vi "oa_Extract XY Signal Segment (2D Array).vi"(0 "XY signals":cluster{"X":dbl[], "Y":dbl[]}[][](array[cluster]) {"X" format="%.2f"; "Y" format="%.2f"}, 1 "X axis selection":u16(ring)=2 items=["Time", "Revolution", "RPM"], 2 "reset? (F)":bool, 5 "trigger indices":T1, 7 "position info in":T2, 11 "error in (no error)":errorcluster, 12 "indices end?":bool) -> (4 "XY signals out":cluster{"X":dbl[], "Y":dbl[]}[][](array[cluster]) {"X" format="%.2f"; "Y" format="%.2f"}, 8 "position info out":T2, 14 "reached end?":bool, 15 "error out":errorcluster)   [LabVIEW 2017, in "SoundVib_OAUtility.lvlib"]
uses:
  <vilib>/addons/Sound and Vibration/Order Analysis/Utility/SoundVib_OAUtility.lvlib
  <vilib>/addons/Sound and Vibration/Order Analysis/Misc/OAT Position Info.ctl
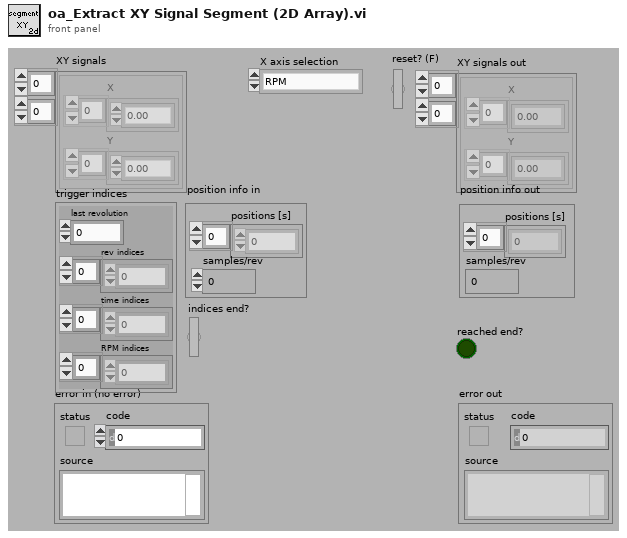
[diagram p1: front panel]
types:
  T1 = cluster{"last revolution":dbl, "rev indices":dbl[], "time indices":dbl[], "RPM indices":dbl[]}
  T2 = typedef "OAT Position Info.ctl" = cluster{"positions [s]":dbl[], "samples/rev":dbl}
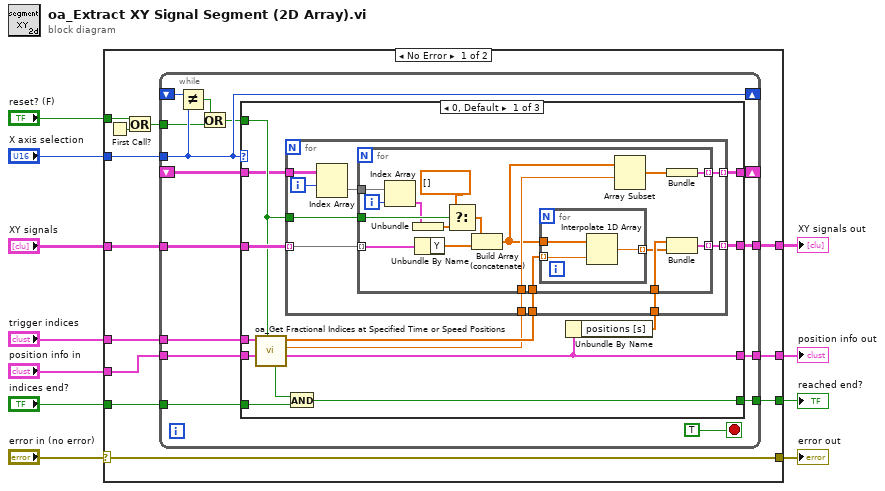
[diagram p0: block diagram]
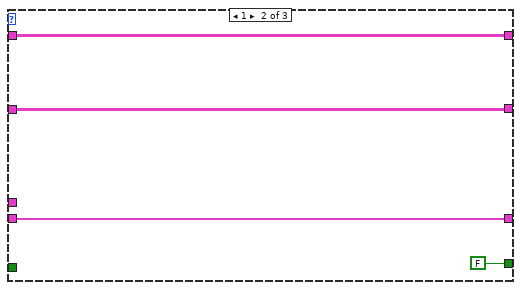
[diagram p2: hidden frame]
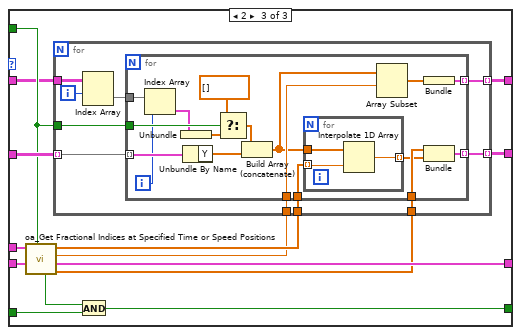
[diagram p3: hidden frame]
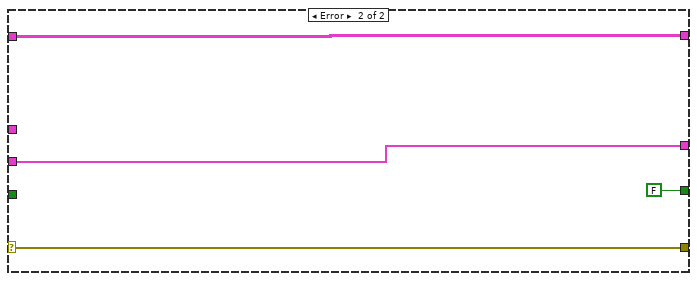
[diagram p4: hidden frame]
diagram:
  n1 = case shown="No Error" "error in (no error)" {
    selector: "error in (no error)" -> [w14 w134]
    tunnel: [w14 w134] -> w10
    tunnel: "reset? (F)" -> [w23 _]
    tunnel: "XY signals" -> [w19 w133]
    tunnel: [w20 w133] -> w7
    tunnel: "position info in" -> [w16 w132]
    tunnel: "trigger indices" -> [w17 _]
    tunnel: "X axis selection" -> [w21 _]
    tunnel: [w15 w132] -> w3
    tunnel: "indices end?" -> [w13 _]
    tunnel: [w12 FALSE] -> w1
    frame No Error {
      n2 = First Call?() -> (First Call?: T/F=w22:bool)
      n3 = Or(x=w23, y=w22) -> (x .or. y?=w18:bool)
      n4 = while {
        tunnel: w21 -> [w29]
        tunnel: [w38] -> w20
        tunnel: w19 -> [w37]
        tunnel: w18 -> [w27]
        tunnel: w17 -> [w36]
        tunnel: w16 -> [w35]
        tunnel: [w34] -> w15
        shift-right: [w32] -> _
        shift-left: _ -> [w31]
        shift-right: [w29] -> _
        shift-left: _ -> [w30]
        tunnel: w13 -> [w25]
        tunnel: [w24] -> w12
        stop <- TRUE stop-if-true
        n5 = Not Equal?(x=w30, y=w29) -> (x != y?=w26:bool)
        n6 = Or(x=w26, y=w27) -> (x .or. y?=w28:bool)
        n7 = case shown="0, Default" w29 {
          tunnel: [w46 w86 w95] -> w38
          tunnel: w37 -> [w50 w86 w98]
          tunnel: w28 -> [w43 _ w97]
          tunnel: w36 -> [w52 _ w94]
          tunnel: w35 -> [w51 w85 w93]
          tunnel: [w48 w85 w92] -> w34
          tunnel: [w44 w84 w96] -> w32
          tunnel: w31 -> [w42 w84 w90]
          tunnel: w25 -> [w41 _ w89]
          tunnel: [w39 FALSE w87] -> w24
          frame 0, Default {
            n8 = call <vilib>:"oa_Get Fractional Indices at Specified Time or Speed Positions.vi"("reset? (F)"=w43, "position info in"=w51, "trigger indices"=w52) -> ("position info out"=w48:T2, "buffer index"=w45:dbl, "fractional indices out"=w49:dbl[], "indices buffer empty?"=w40:bool)  [unwired: 4 in, 1 out]
            n9 = And(x=w40, y=w41) -> (x .and. y?=w39:bool)
            n10 = Unbundle By Name(w48) -> ("positions [s]"=w47:dbl[])
            n11 = for {
              tunnel: w50 -> [w62] mode=indexing
              tunnel: w49 -> [w61]
              tunnel: w47 -> [w60]
              tunnel: [w59] -> w46 mode=indexing
              tunnel: w45 -> [w58]
              tunnel: [w57] -> w44 mode=indexing
              tunnel: w43 -> [w56]
              tunnel: w42 -> [w55]
              i -> [w54]
              n12 = Index Array(array=w55, index (row)=w54) -> (element=w53:cluster{dbl[]}[])  [unwired: 1 in]
              n13 = for {
                tunnel: w62 -> [w79] mode=indexing
                tunnel: w61 -> [w78]
                tunnel: w60 -> [w77]
                tunnel: [w76] -> w59 mode=indexing
                tunnel: w58 -> [w75]
                tunnel: [w74] -> w57 mode=indexing
                tunnel: w56 -> [w73]
                tunnel: w53 -> [w65]
                i -> [w63]
                n14 = Index Array(array=w65, index=w63) -> (element=w64:cluster{dbl[]})
                n15 = Unbundle(w64) -> (w70:dbl[])
                n16 = Unbundle By Name(w79) -> ("Y"=w68:dbl[])
                n17 = Select(t=dbl[] [], s=w73, f=w70) -> (s? t:f=w69:dbl[])
                n18 = Build Array (concatenate)(w69, w68) -> (w67:dbl[])
                n19 = for {
                  tunnel: w67 -> [w82]
                  tunnel: w78 -> [w81] mode=indexing
                  tunnel: [w80] -> w72 mode=indexing
                  n20 = Interpolate 1D Array(1:w81, 2:w82) -> (0:w80:dbl)
                }
                n21 = Array Subset(array=w67, index=w75) -> (w71:dbl[])  [unwired: 1 in]
                n22 = Bundle(w71) -> (w74:cluster{dbl[]})  [unwired: 1 in]
                n23 = Bundle("positions [s]"=w77, w72) -> (w76:cluster{"positions [s]":dbl[], dbl[]})  [unwired: 1 in]
              }
            }
          }
          frame 1 {
          }
          frame 2 {
            n24 = call <vilib>:"oa_Get Fractional Indices at Specified Time or Speed Positions.vi"("reset? (F)"=w97, "position info in"=w93, "trigger indices"=w94) -> ("rpm indices"=w91:dbl[], "position info out"=w92:T2, "buffer index"=w99:dbl, "fractional indices out"=w100:dbl[], "indices buffer empty?"=w88:bool)  [unwired: 4 in]
            n25 = for {
              tunnel: w100 -> [w110]
              tunnel: w99 -> [w109]
              tunnel: w98 -> [w108] mode=indexing
              tunnel: w97 -> [w107]
              tunnel: [w106] -> w96 mode=indexing
              tunnel: [w105] -> w95 mode=indexing
              tunnel: w91 -> [w104]
              tunnel: w90 -> [w103]
              i -> [w102]
              n26 = Index Array(array=w103, index (row)=w102) -> (element=w101:cluster{dbl[]}[])  [unwired: 1 in]
              n27 = for {
                tunnel: w110 -> [w127]
                tunnel: w109 -> [w126]
                tunnel: w108 -> [w125] mode=indexing
                tunnel: w107 -> [w124]
                tunnel: [w123] -> w106 mode=indexing
                tunnel: [w122] -> w105 mode=indexing
                tunnel: w104 -> [w121]
                tunnel: w101 -> [w113]
                i -> [w111]
                n28 = Index Array(array=w113, index=w111) -> (element=w112:cluster{dbl[]})
                n29 = Unbundle(w112) -> (w118:dbl[])
                n30 = Unbundle By Name(w125) -> ("Y"=w115:dbl[])
                n31 = Select(t=dbl[] [], s=w124, f=w118) -> (s? t:f=w116:dbl[])
                n32 = Build Array (concatenate)(w116, w115) -> (w114:dbl[])
                n33 = for {
                  tunnel: w114 -> [w130]
                  tunnel: w127 -> [w129] mode=indexing
                  tunnel: [w128] -> w120 mode=indexing
                  n34 = Interpolate 1D Array(1:w129, 2:w130) -> (0:w128:dbl)
                }
                n35 = Array Subset(array=w114, index=w126) -> (w119:dbl[])  [unwired: 1 in]
                n36 = Bundle(w119) -> (w123:cluster{dbl[]})  [unwired: 1 in]
                n37 = Bundle("rpm indices"=w121, w120) -> (w122:cluster{"rpm indices":dbl[], dbl[]})  [unwired: 1 in]
              }
            }
            n38 = And(x=w88, y=w89) -> (x .and. y?=w87:bool)
          }
        }
      }
    }
    frame Error {
    }
  }
  "error out" <- w10
  "XY signals out" <- w7
  "position info out" <- w3
  "reached end?" <- w1
